vi "GetQRcode.vi"(0 "自动？":enum16{"禁止自适应版本", "自适应版本"}(ring)=enum."自适应版本", 1 "图片尺寸":T1, 5 "纠错等级":u16(ring)=2 items=["L(7%)", "M(15%)", "Q(25%)", "H(30%)"], 7 "版本":u16(ring)=1 items=["1"=1, "2"=2, "3"=3, "4"=4, "5"=5, "6"=6, "7"=7, "8"=8, "9"=9, "10"=10, "11"=11, "12"=12, "13"=13, "14"=14, "15"=15, "16"=16, "17"=17, "18"=18, "19"=19, "20"=20, "21"=21, "22"=22, "23"=23, "24"=24, "25"=25, "26"=26, "27"=27, "28"=28, "29"=29, "30"=30, "31"=31, "32"=32, "33"=33, "34"=34, "35"=35, "36"=36, "37"=37, "38"=38, "39"=39, "40"=40], 9 "掩模图形":u16(ring) items=["000", "001", "010", "011", "100", "101", "110", "111"], 11 "输入文本":string="殷培\n2013年9月5日\nemail:yin-pei@qq.com", 12 "边界距离":cluster{"x":i16, "y":i16}) -> (4 "二维码":bool[][](array[boolean]), 6 "显示起点":cluster{dbl, dbl}, 8 "像素大小":cluster{dbl, dbl}, 10 "扩展版本":i32)   [LabVIEW 2016, in "opSignIn.lvlib"]
uses:
  opSignIn.lvlib
  <vilib>/Utility/miscctls.llb/LVBoundsTypeDef.ctl
  QR_ENCODE/QR_ENCODE.lvlib
panel:
  out "p_len_m":i32
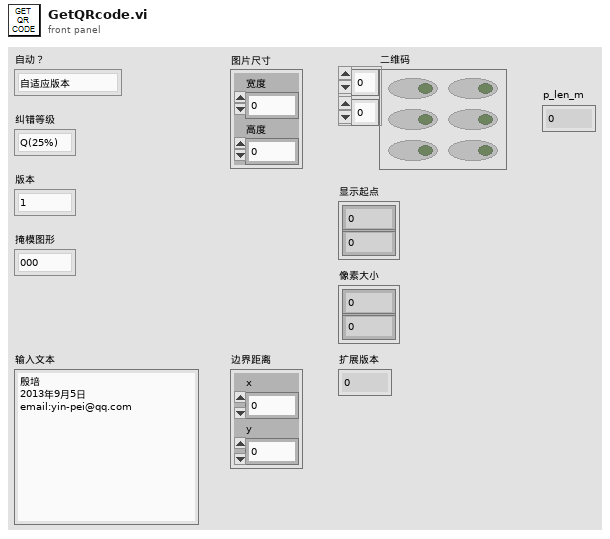
[diagram p1: front panel]
types:
  T1 = typedef "LVBoundsTypeDef.ctl" = cluster{"Width":u32, "Height":u32}
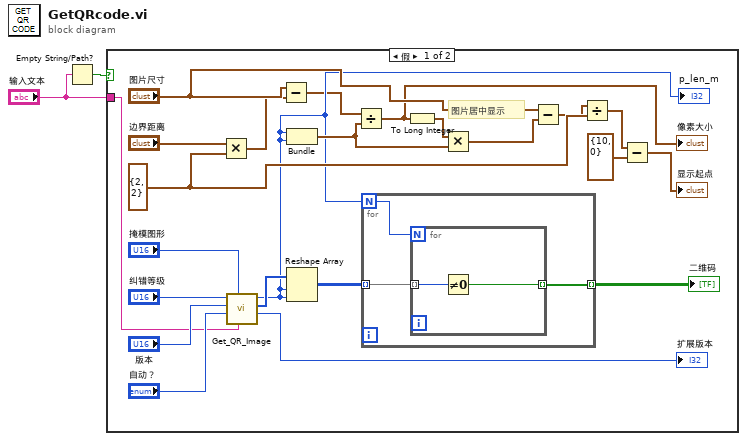
[diagram p0: block diagram]
diagram:
  n1 = Empty String/Path?(string/path="输入文本") -> (empty?=w1:bool)
  n2 = case shown="假" w1 {
    tunnel: "输入文本" -> [w3 _]
    frame False {
      w23 = cluster{"x":i16, "y":i16} {"x"=2, "y"=2} ("y")
      # "图片居中显示"
      n3 = Multiply(x="边界距离", y=w23) -> (x*y=w12:cluster{"x":i16, "y":i16})
      n4 = call "Get_QR_Image.vi"("strEncodeData"=w3, "nMaskingNo"="掩模图形", "bAutoExtent"="自动？", "nVersion"="版本", "nLevel"="纠错等级") -> ("p_nVersion"=→"扩展版本":i32, "p_buf"=w13:i8[], "p_len_m"=w11:i32)  [unwired: 3 in, 1 out]
      "p_len_m" <- w11
      n5 = Subtract(x="图片尺寸", y=w12) -> (x-y=w10:T1)
      n6 = Bundle("p_len_m"=w11, "p_len_m"=w11) -> (w19:cluster{"p_len_m":i32, "p_len_m":i32})  [unwired: 1 in]
      n7 = Reshape Array(w13, w11, w11) -> (w14:i8[][])
      n8 = Divide(x=w10, y=w19) -> (x/y=w8:cluster{dbl, dbl})
      "像素大小" <- w8
      n9 = for {
        N: w11 -> [w26]
        tunnel: w14 -> [w28] mode=indexing
        tunnel: [w27] -> w15 mode=indexing
        n10 = for {
          N: w26 -> [_]
          tunnel: w28 -> [w30] mode=indexing
          tunnel: [w29] -> w27 mode=indexing
          n11 = Not Equal To 0?(x=w30) -> (x != 0?=w29:bool)
        }
      }
      "二维码" <- w15
      n12 = To Long Integer(number=w8) -> (32bit integer=w18:cluster{i32, i32})
      n13 = Multiply(x=w18, y=w19) -> (x*y=w21:cluster{i32, i32})
      n14 = Subtract(x="图片尺寸", y=w21) -> (x-y=w22:T1)
      n15 = Divide(x=w22, y=w23) -> (x/y=w25:cluster{dbl, dbl})
      n16 = Subtract(x=w25, y=cluster{"x":i16, "y":i16} {"x"=10, "y"=0} ("point(x,y)")) -> (x-y=→"显示起点":cluster{dbl, dbl})
    }
    frame True {
    }
  }
